vi "Get Motor Status.vi"(7 "error in (no error)":errorcluster, 10 "VISA in":refnum<visa-resource-name>) -> (0 "error out":errorcluster, 2 "Motors Busy?":bool, 3 "VISA out":refnum<visa-resource-name>)   [LabVIEW 2018, in "ASI TG-1000.lvlib"]
doc: "Checks whether the motors are running; the equivalent of using the STATUS command."
uses:
  ASI TG-1000.lvlib
  Utility/Serial Response Syntax.ctl
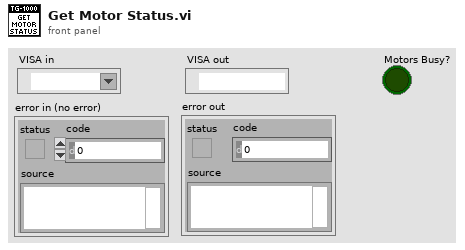
[diagram p1: front panel]
types:
  T1 = typedef "ASI TG-1000.lvlib/Serial Response Syntax.ctl" = enum16{":A then single line", "Single line, no :A", ":A or : then single line", ":A then single number", ":A or : then single number", ":A then <axis>= single number"}
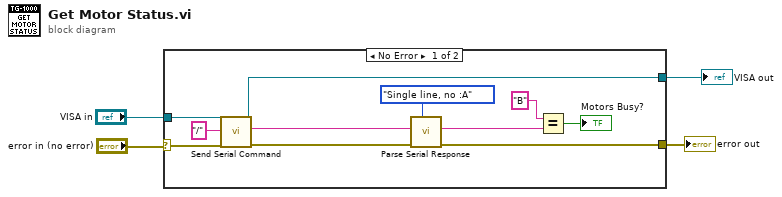
[diagram p0: block diagram]
diagram:
  n1 = case shown="No Error" "error in (no error)" {
    selector: "error in (no error)" -> [w5 w17]
    tunnel: "VISA in" -> [w15 w16]
    tunnel: [w14 w16] -> w3
    tunnel: [w6 w17] -> w2
    frame No Error {
      n2 = call "Send Serial Command.vi"("error in (no error)"=w5, "Command"="/", "VISA in"=w15) -> ("error out"=w7:errorcluster, "Response"=w10:string, "VISA out"=w14:refnum<visa-resource-name>)  [unwired: 6 in]
      n3 = call "Parse Serial Response.vi"("Response Syntax"=Serial_Response_Syntax."Single line, no :A", "error in (no error)"=w7, "Raw Response"=w10) -> ("error out"=w6:errorcluster, "Parsed String"=w8:string)  [unwired: 5 in, 2 out]
      n4 = Equal?(x="B" ("y"), y=w8) -> (x = y?=→"Motors Busy?":bool)
    }
    frame Error {
    }
  }
  "VISA out" <- w3
  "error out" <- w2
